vi "Array.vi"(5 "Array":string[](array[string]), 7 "Boolean":bool, 9 "String":string) -> (6 "Array":string[](array[string]))   [LabVIEW 2014, in "FH 55.lvlib"]
doc: "Am Display wird immer nur eine aktive Funktion angezeigt (Max_Display, Temp_Display oder Relative-Funktion). Dieses Array gibt die reihenfolge an, in welcher die Funktionen am Display angezeigt werden\n\nOn display will be only one active function display (Max_Display, Temp_Display or Relative function). This array is the order in which the functions are displayed on the display"
uses:
  FH 55.lvlib
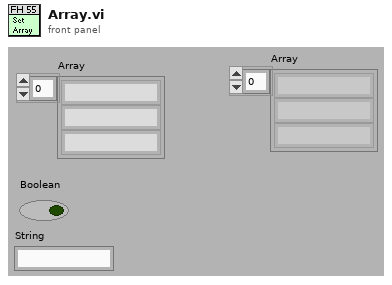
[diagram p1: front panel]
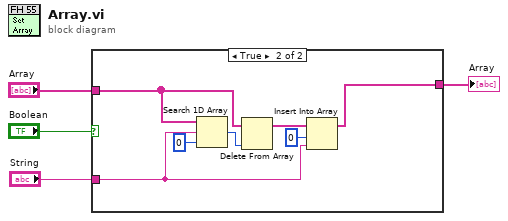
[diagram p0: block diagram]
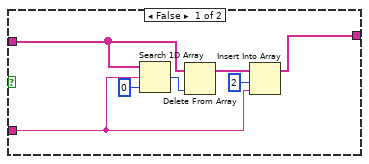
[diagram p2: hidden frame]
diagram:
  n1 = case shown="True" "Boolean" {
    tunnel: "Array" -> [w7 w13]
    tunnel: "String" -> [w5 w14]
    tunnel: [w6 w12] -> w1
    frame False {
      n2 = Search 1D Array(1D array=w7, element=w5, start index (0)=0) -> (index of element=w10:i32)
      n3 = Delete From Array(array=w7, index=w10) -> (array with subset deleted=w8:string[])  [unwired: 1 in, 1 out]
      n4 = Insert Into Array(array=w8, index=2, new element=w5) -> (w6:string[])
    }
    frame True {
      n5 = Search 1D Array(1D array=w13, element=w14, start index (0)=0) -> (index of element=w17:i32)
      n6 = Delete From Array(array=w13, index=w17) -> (array with subset deleted=w15:string[])  [unwired: 1 in, 1 out]
      n7 = Insert Into Array(array=w15, index=0, new element=w14) -> (w12:string[])
    }
  }
  "Array" <- w1
